vi "Index From GUID.vi"(8 "error in":errorcluster, 9 "GUID":string, 11 "Objects In":refnum<class "ObjectSettings.lvclass">[](array[class])) -> (0 "error out":errorcluster, 1 "Index":i32, 2 "Object Setting Out":refnum<class "ObjectSettings.lvclass">, 3 "Objects Out":refnum<class "ObjectSettings.lvclass">[](array[class]))   [LabVIEW 2019, in "Setting Database.lvclass"]
uses:
  Setting Database.lvclass
  ObjectSettings/ObjectSettings.lvclass
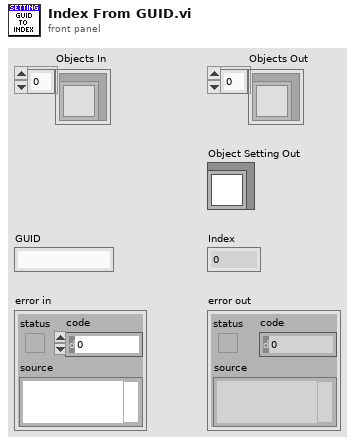
[diagram p1: front panel]
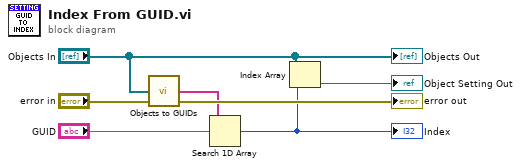
[diagram p0: block diagram]
diagram:
  n1 = call "Objects to GUIDs.vi"("error in (no error)"="error in", "Objects"="Objects In") -> ("error out"=→"error out":errorcluster, "GUIDs"=w5:string[])  [unwired: 2 in]
  n2 = Search 1D Array(1D array=w5, element="GUID") -> (index of element=w1:i32)  [unwired: 1 in]
  "Index" <- w1
  n3 = Index Array(array="Objects In", index=w1) -> (element=→"Object Setting Out":refnum<class "ObjectSettings.lvclass">)
  "Objects Out" <- "Objects In"
